vi "Create_Preview.vi"(0 "vi reference":refnum<vi>, 11 "error in (no error)":errorcluster) -> (4 "vi reference out":refnum<vi>, 15 "error out":errorcluster)   [LabVIEW 2018, in "NISAST VI Scripting.lvlib" / "VI.lvlib" / "Connector.lvlib"]
uses:
  Connector.lvlib
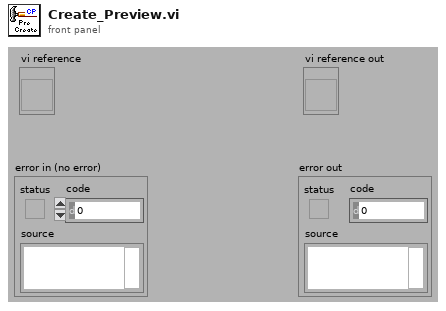
[diagram p1: front panel]
types:
  T1 = typedef "NISAST VI Scripting.lvlib/VI.lvlib/Front Panel.lvlib/Connector Pane Type.ctl" = enum16{"4-2-2-4", "5-2-2-2-5", "Others"}
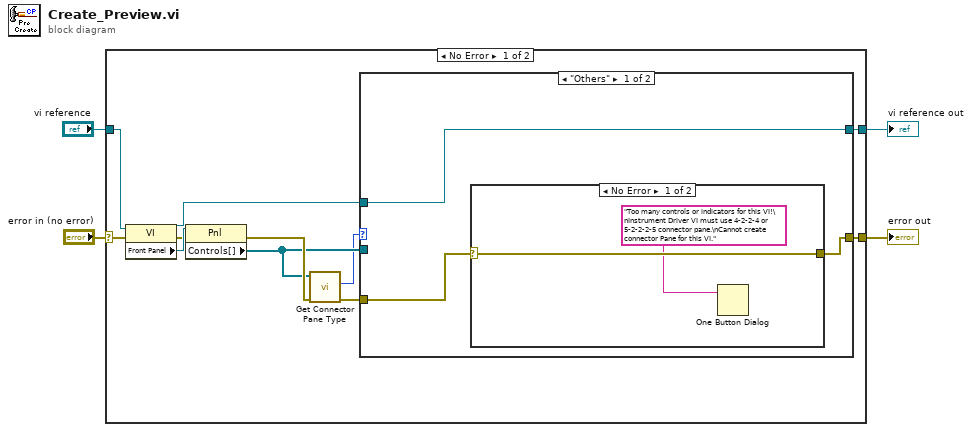
[diagram p0: block diagram]
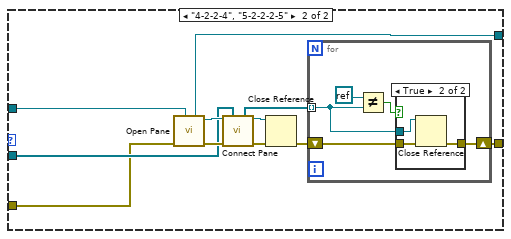
[diagram p3: hidden frame]
diagram:
  n1 = case shown="No Error" "error in (no error)" {
    selector: "error in (no error)" -> [w12 w43]
    tunnel: [w10 w43] -> w2
    tunnel: "vi reference" -> [w13 w42]
    tunnel: [w9 w42] -> w1
    frame No Error {
      n2 = property class="VI"(reference=w13, error in=w12) -> (reference out=w11:refnum<vi>, error out=w14:errorcluster, "Front Panel"=w15:refnum<vi>)
      n3 = property class="Pnl"(reference=w15, error in=w14) -> (error out=w8:errorcluster, "Controls[]"=w7:refnum<vi>[])  [unwired: 1 out]
      n4 = call "Get Connector Pane Type.vi"("error in (no error)"=w8, "Controls[]"=w7) -> ("error out"=w6:errorcluster, "Connector Pane Type"=w5:T1)  [unwired: 7 out]
      n5 = case shown="\"Others\"" w5 {
        tunnel: w11 -> [w18 w28]
        tunnel: [w16 w25] -> w10
        tunnel: [w18 w24] -> w9
        tunnel: w7 -> [_ w23]
        tunnel: w6 -> [w17 w22]
        frame "Others" {
          n6 = case shown="No Error" w17 {
            selector: w17 -> [w20 w21]
            tunnel: [w20 w21] -> w16
            frame No Error {
              n7 = One Button Dialog(message="Too many controls or indicators for this VI!\nInstrument Driver VI must use 4-2-2-4 or 5-2-2-2-5 connector pane.\nCannot create connector Pane for this VI.") -> ()  [unwired: 2 out]
            }
            frame Error {
            }
          }
        }
        frame "4-2-2-4", "5-2-2-2-5" {
          n8 = call "Open Pane.vi"("vi refnum"=w28, "error in"=w22) -> ("error out"=w29:errorcluster, "connect pane"=w32:refnum<vi>, "vi refnum out"=w24:refnum<vi>)  [unwired: 7 out]
          n9 = call "Connect Pane.vi"("connect pane"=w32, "Controls[]"=w23, "error in"=w29) -> ("Controls[] output"=w26:refnum<vi>[], "connect pane out"=w31:refnum<vi>, "error out"=w30:errorcluster)  [unwired: 10 out]
          n10 = Close Reference(reference=w31, error in (no error)=w30) -> (error out=w27:errorcluster)
          n11 = for {
            shift-right: [w36] -> w25
            shift-left: w27 -> [w37]
            tunnel: w26 -> [w34] mode=indexing
            n12 = Not Equal?(x=refnum<k0> refnum, y=w34) -> (x != y?=w33:bool)
            n13 = case shown="True" w33 {
              tunnel: w37 -> [w38 w41]
              tunnel: [w38 w40] -> w36
              tunnel: w34 -> [_ w39]
              frame False {
              }
              frame True {
                n14 = Close Reference(reference=w39, error in (no error)=w41) -> (error out=w40:errorcluster)
              }
            }
          }
        }
      }
    }
    frame Error {
    }
  }
  "error out" <- w2
  "vi reference out" <- w1
